vi "Do Create Control.vi"(8 "error in (no error)":errorcluster, 10 "create_control Argument":T3, 11 "Data Cluster in":T1) -> (0 "error out":errorcluster, 2 "new reference":i32, 3 "Data Cluster out":T1)   [LabVIEW 2025, in "Scripting Server.lvlib"]
uses:
  Scripting Server.lvlib
  create_control Argument--cluster.ctl
  create_control (Reply Payload)--cluster.ctl
  Module Data--cluster.ctl
  Config Data.ctl
  Tools/Tools.lvlib
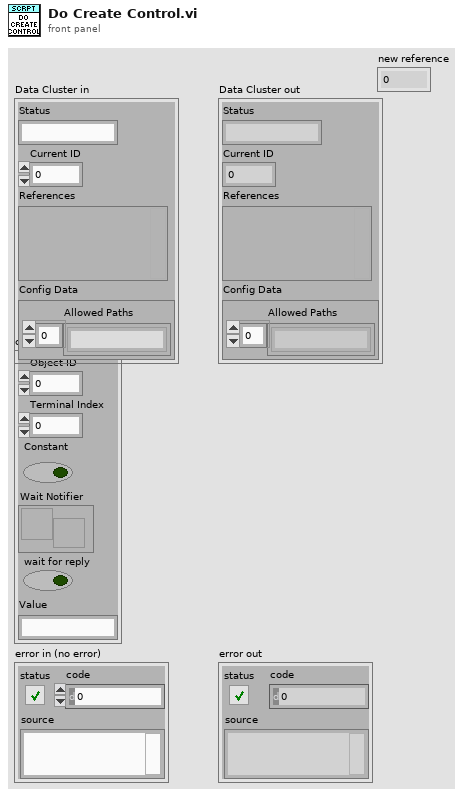
[diagram p1: front panel]
types:
  T1 = typedef "Scripting Server.lvlib/Module Data--cluster.ctl" = cluster{"Status":string, "Current ID":i32, "References":variant, "Config Data":T2}
  T2 = typedef "Scripting Server.lvlib/Config Data.ctl" = cluster{"Allowed Paths":string[]}
  T3 = typedef "Scripting Server.lvlib/create_control Argument--cluster.ctl" = cluster{"Object ID":i32, "Terminal Index":i32, "Constant":bool, "Wait Notifier":refnum<notifier>, "wait for reply":bool, "Value":string}
  T4 = typedef "Scripting Server.lvlib/Tools.lvlib/Datatypes.ctl" = enum16{"Float", "Int", "String", "String Array", "Int Array", "Float Array", "Bool Array", "Bool", "Invalid"}
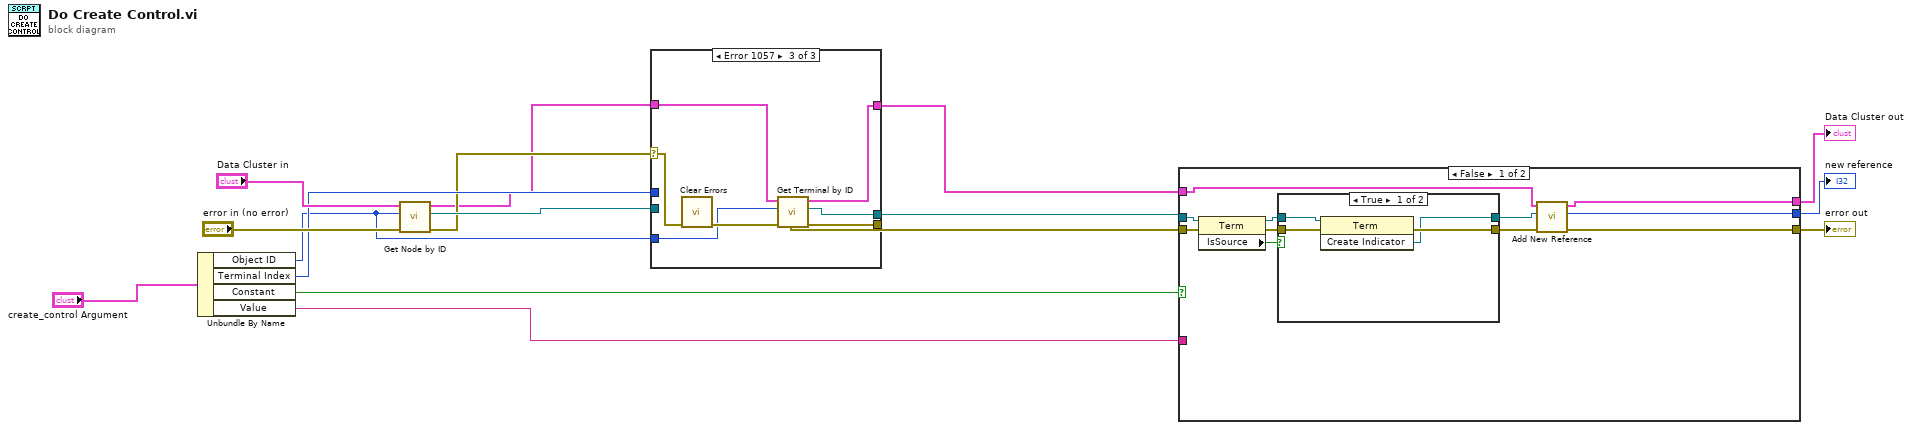
[diagram p0: block diagram]
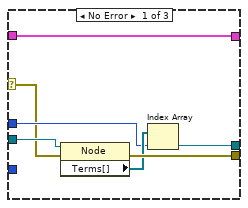
[diagram p2: hidden frame]
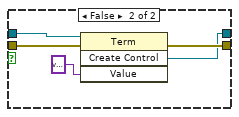
[diagram p4: hidden frame]
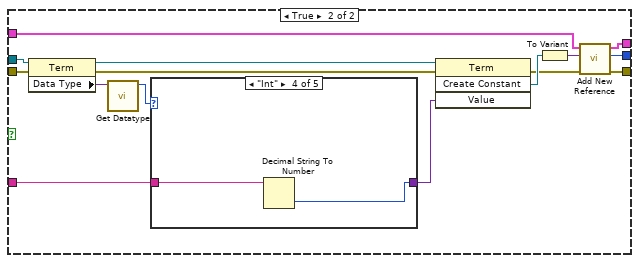
[diagram p5: hidden frame]
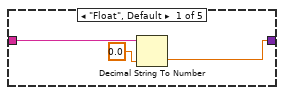
[diagram p6: hidden frame]
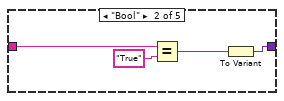
[diagram p7: hidden frame]
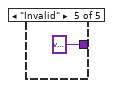
[diagram p9: hidden frame]
diagram:
  n1 = Unbundle By Name("create_control Argument") -> ("Object ID"=w1:i32, "Terminal Index"=w12:i32, "Constant"=w9:bool, "Value"=w6:string)
  n2 = call "Get Node by ID.vi"("error in (no error)"="error in (no error)", "ID"=w1, "Data Cluster in"="Data Cluster in") -> ("error out"=w4:errorcluster, "specific class reference"=w5:refnum<vi>, "Data Cluster out"=w3:T1)  [unwired: 6 in]
  n3 = case shown="Error 1057" w4 {
    selector: w4 -> [w18 w25 w32]
    tunnel: [w23 w25 w30] -> w13
    tunnel: w12 -> [w21 _ _]
    tunnel: [w20 _ w26] -> w10
    tunnel: w5 -> [w19 _ _]
    tunnel: w3 -> [w17 w24 w29]
    tunnel: [w17 w24 w28] -> w2
    tunnel: w1 -> [_ _ w27]
    frame No Error {
      n4 = property class="Node"(reference=w19, error in=w18) -> (error out=w23:errorcluster, "Terms[]"=w22:refnum<vi>[])  [unwired: 1 out]
      n5 = Index Array(array=w22, index=w21) -> (element=w20:refnum<vi>)
    }
    frame Default {
    }
    frame Error {
      n6 = call <vilib>:"Clear Errors.vi"("error in (no error)"=w32) -> ("error out"=w31:errorcluster)  [unwired: 5 in, 1 out]
      n7 = call "Get Terminal by ID.vi"("error in (no error)"=w31, "ID"=w27, "Data Cluster in"=w29) -> ("error out"=w30:errorcluster, "specific class reference"=w26:refnum<vi>, "Data Cluster out"=w28:T1)  [unwired: 6 in]
    }
  }
  n8 = case shown="False" w9 {
    tunnel: w13 -> [w43 w67]
    tunnel: [w37 w61] -> w11
    tunnel: w10 -> [w41 w58]
    tunnel: [w36 w66] -> w8
    tunnel: w2 -> [w35 w65]
    tunnel: [w33 w60] -> w7
    tunnel: w6 -> [_ w55]
    frame False {
      n9 = property class="Term"(reference=w41, error in=w43) -> (reference out=w40:refnum<vi>, error out=w42:errorcluster, "IsSource"=w39:bool)
      n10 = case shown="True" w39 {
        tunnel: [w47 w52] -> w38
        tunnel: w42 -> [w46 w51]
        tunnel: w40 -> [w45 w50]
        tunnel: [w44 w49] -> w34
        frame True {
          n11 = invoke class="Term" method="Create Indicator"(reference=w45, error in=w46) -> (error out=w47:errorcluster, "Create Indicator"=w44:refnum<vi>)  [unwired: 1 in, 1 out]
        }
        frame False {
          n12 = invoke class="Term" method="Create Control"(reference=w50, error in=w51, "Value"=variant) -> (error out=w52:errorcluster, "Create Control"=w49:refnum<vi>)  [unwired: 1 in, 2 out]
        }
      }
      n13 = call "Add New Reference.vi"("error in (no error)"=w38, "Variant"=w34, "Data Cluster in"=w35) -> ("error out"=w37:errorcluster, "new reference"=w33:i32, "Data Cluster out 2"=w36:T1)  [unwired: 6 in]
    }
    frame True {
      n14 = property class="Term"(reference=w58, error in=w67) -> (reference out=w57:refnum<vi>, error out=w59:errorcluster, "Data Type"=w56:variant)
      n15 = call "Get Datatype.vi"("Value"=w56) -> ("datatypes"=w53:T4)  [unwired: 10 in]
      n16 = case shown="\"Int\"" w53 {
        tunnel: w55 -> [w70 w73 w75 w77 _]
        tunnel: [w68 w71 w75 w76 variant ("Variant")] -> w54
        frame "Float", Default {
          n17 = Decimal String To Number(string=w70, default (0L)=0.0 ("default (0 I32)")) -> (number=w68:dbl)  [unwired: 1 in, 1 out]
        }
        frame "Bool" {
          n18 = Equal?(x=w73, y="True") -> (x = y?=w72:bool)
          n19 = To Variant(anything=w72) -> (Variant=w71:variant)
        }
        frame "String" {
        }
        frame "Int" {
          n20 = Decimal String To Number(string=w77) -> (number=w76:i32)  [unwired: 2 in, 1 out]
        }
        frame "Invalid" {
        }
      }
      n21 = invoke class="Term" method="Create Constant"(reference=w57, error in=w59, "Value"=w54) -> (error out=w62:errorcluster, "Create Constant"=w64:refnum<vi>)  [unwired: 1 in, 2 out]
      n22 = To Variant(anything=w64) -> (Variant=w63:variant)
      n23 = call "Add New Reference.vi"("error in (no error)"=w62, "Variant"=w63, "Data Cluster in"=w65) -> ("error out"=w61:errorcluster, "new reference"=w60:i32, "Data Cluster out 2"=w66:T1)  [unwired: 6 in]
    }
  }
  "Data Cluster out" <- w8
  "error out" <- w11
  "new reference" <- w7
